vi "Get Result Color.vi"(1 "Result":T1) -> (0 "Color":string)   [LabVIEW 2015, in "HtmlReportPlugin.lvclass"]
uses:
  HtmlReportPlugin.lvclass
  Core/Step/STEP_STATUS.ctl
  Core/Step.lvclass
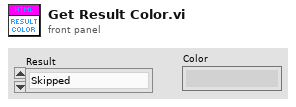
[diagram p1: front panel]
types:
  T1 = typedef "Step.lvclass/STEP_STATUS.ctl" = enum16{"Skipped", "Done", "Passed", "Failed", "Error"}
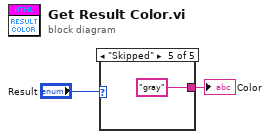
[diagram p0: block diagram]
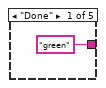
[diagram p2: hidden frame]
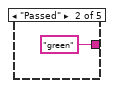
[diagram p3: hidden frame]
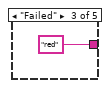
[diagram p4: hidden frame]
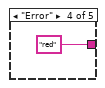
[diagram p5: hidden frame]
diagram:
  n1 = case shown="\"Skipped\"" "Result" {
    tunnel: ["green" "green" "red" "red" "gray"] -> w1
    frame "Done" {
    }
    frame "Passed" {
    }
    frame "Failed" {
    }
    frame "Error" {
    }
    frame "Skipped" {
    }
  }
  "Color" <- w1
